vi "ParseSQLOperatorResults.vi"(11 "Basic Info":T1[](array[typedef])) -> (3 "Array":cluster{"Full Name":string, "Numeric":i32}[](array[cluster]))   [LabVIEW 2018]
uses:
  OSTEP_MySQLdBTools/TypeDefs/BasicOperatorInfo.ctl
  OSTEP_MySQLdBTools/MySQLTools.lvlib
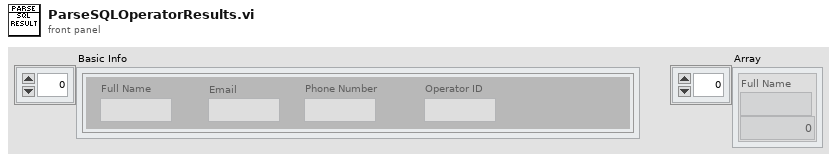
[diagram p1: front panel]
types:
  T1 = typedef "MySQLTools.lvlib/BasicOperatorInfo.ctl" = cluster{"Full Name":string, "Email":string, "Phone Number":string, "Operator ID":string}
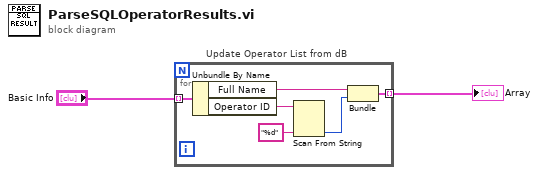
[diagram p0: block diagram]
diagram:
  n1 = for "Update Operator List from dB" {
    tunnel: "Basic Info" -> [w8] mode=indexing
    tunnel: [w4] -> w2 mode=indexing
    n2 = Unbundle By Name(w8) -> ("Full Name"=w5:string, "Operator ID"=w7:string)
    n3 = Scan From String(format string="%d", input string=w7) -> (output 1=w3:i32)  [unwired: 3 in, 3 out]
    n4 = Bundle("Full Name"=w5, w3) -> (w4:cluster{"Full Name":string, i32})  [unwired: 1 in]
  }
  "Array" <- w2
